vi "Periodic Tasks (Austen Adler's conflicted copy 2013-10-16).vi"(8 "error in":errorcluster) -> ()   [LabVIEW 2012]
doc: "This VI runs in parallel to other tasks. It can contain as many user-defined periodic loops as you need. These can carry out PID or other sorts of timed response."
uses:
  <vilib>/Rock Robotics/SystemInterfaces/Utilities/FPGA_UtilitiesLED Source.ctl
  <vilib>/Rock Robotics/SystemInterfaces/Utilities/FPGA_UtilitiesLED State.ctl
  <vilib>/Rock Robotics/WPI/Compressor/WPI_CompressorGetSetRefNum.vi
  <vilib>/Rock Robotics/WPI/Joystick/WPI_JoystickGetSetRefNum.vi
  Robot Global Data.vi
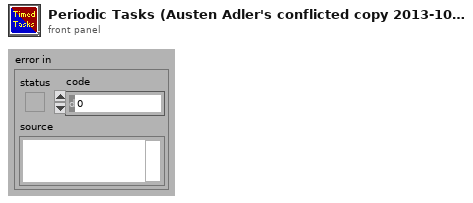
[diagram p1: front panel]
types:
  T1 = typedef "FPGA_UtilitiesLED State.ctl" = enum16{"Off", "On", "Toggle"}
  T2 = typedef "FPGA_UtilitiesLED Source.ctl" = enum16{"User LED", "FPGA LED"}
  T3 = typedef "WPI_JoystickDevRef.ctl" = cluster{"Device":T4}
  T4 = typedef "WPI_JoystickDeviceEnum.ctl" = enum16{"USB 1", "USB 2", "USB 3", "USB 4", "Kinect 1", "Kinect 2"}
  T5 = typedef "WPI_JoystickButtonState.ctl" = cluster{"Button 1":bool, "Button 2":bool, "Button 3":bool, "Button 4":bool, "Button 5":bool, "Button 6":bool, "Button 7":bool, "Button 8":bool, "Button 9":bool, "Button 10":bool, "Button 11":bool, "Button 12":bool}
  T6 = typedef "WPI_CompressorDevRef.ctl" = cluster{"DevStatus":errorcluster, "DigitalInputDevRef":T7, "RelayDevRef":T10}
  T7 = typedef "WPI_DigitalInputDevRef.ctl" = cluster{"DevStatus":errorcluster, "DIO Channel":T8, "Digital Module":T9}
  T8 = typedef "FPGA_DIOChannel.ctl" = enum8{"DIO 1", "DIO 2", "DIO 3", "DIO 4", "DIO 5", "DIO 6", "DIO 7", "DIO 8", "DIO 9", "DIO 10", "DIO 11", "DIO 12", "DIO 13", "DIO 14", "Invalid"}
  T9 = typedef "FPGA_TypedefDigitalModule.ctl" = enum16{"Digital Module 1", "Digital Module 2"}
  T10 = typedef "WPI_RelayDevRef.ctl" = cluster{"DevStatus":errorcluster, "Relay Channel":T11, "Digital Module":T9, "Relay Direction":T12}
  T11 = typedef "FPGA_DIORelayChannel.ctl" = enum8{"Relay 1", "Relay 2", "Relay 3", "Relay 4", "Relay 5", "Relay 6", "Relay 7", "Relay 8", "Invalid"}
  T12 = typedef "WPI_RelayDirection.ctl" = enum16{"Both directions", "Forward only", "Reverse only"}
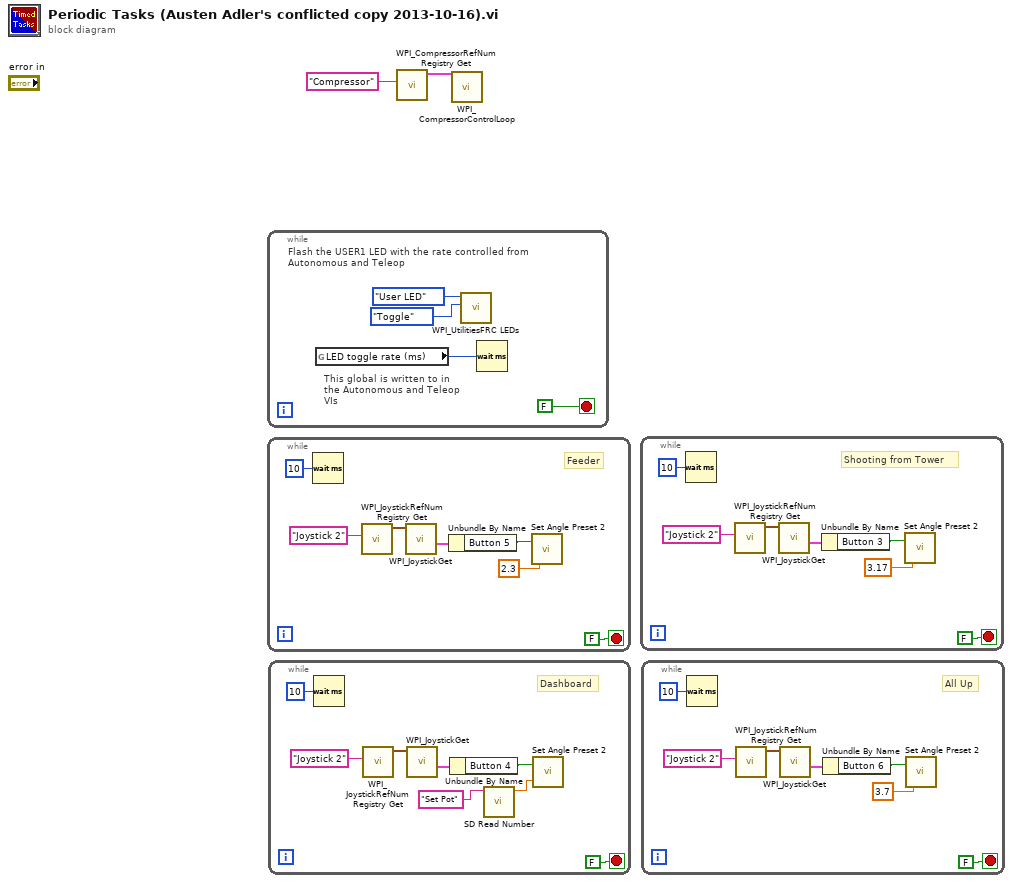
[diagram p0: block diagram]
diagram:
  n1 = while {
    stop <- FALSE stop-if-true
    # "This global is written to in the Autonomous and Teleop VIs"
    # "Flash the USER1 LED with the rate controlled from Autonomous and Teleop"
    n2 = global read "Robot Global Data.vi" "LED toggle rate (ms)"() -> (w3:u32)
    n3 = call <vilib>:"WPI_UtilitiesFRC LEDs.vi"("State"=FPGA_UtilitiesLED_State."Toggle", "LED Type"=FPGA_UtilitiesLED_Source."User LED") -> ()  [unwired: 1 in, 9 out]
    n4 = Wait (ms)(milliseconds to wait=w3) -> ()  [unwired: 1 out]
  }
  n5 = while {
    stop <- FALSE stop-if-true
    # "Feeder"
    n6 = Wait (ms)(milliseconds to wait=u32 10) -> ()  [unwired: 1 out]
    n7 = call <vilib>:"WPI_JoystickRefNum Registry Get.vi"("refnum name"="Joystick 2") -> ("JoystickDevRef"=w13:T3)  [unwired: 1 in, 9 out]
    n8 = call <vilib>:"WPI_JoystickGet.vi"("JoystickDevRef"=w13) -> ("Buttons"=w10:T5)  [unwired: 1 in, 5 out]
    n9 = Unbundle By Name(w10) -> ("Button 5"=w8:bool)
    n10 = call "Set Angle Preset 2.vi"("Set Angle"=2.3, "Enable"=w8) -> ()  [unwired: 1 in]
  }
  n11 = while {
    stop <- FALSE stop-if-true
    # "Dashboard"
    n12 = Wait (ms)(milliseconds to wait=u32 10) -> ()  [unwired: 1 out]
    n13 = call <vilib>:"WPI_JoystickRefNum Registry Get.vi"("refnum name"="Joystick 2") -> ("JoystickDevRef"=w21:T3)  [unwired: 1 in, 9 out]
    n14 = call <vilib>:"WPI_JoystickGet.vi"("JoystickDevRef"=w21) -> ("Buttons"=w18:T5)  [unwired: 1 in, 5 out]
    n15 = Unbundle By Name(w18) -> ("Button 4"=w16:bool)
    n16 = call <vilib>:"SD Read Number.vi"("Name"="Set Pot" ("refnum name")) -> ("Numeric"=w14:dbl)  [unwired: 8 in, 2 out]
    n17 = call "Set Angle Preset 2.vi"("Set Angle"=w14, "Enable"=w16) -> ()  [unwired: 1 in]
  }
  n18 = call <vilib>:"WPI_CompressorRefNum Registry Get.vi"("refnum name"="Compressor") -> ("CompressorDevRef"=w1:T6)  [unwired: 9 in, 1 out]
  n19 = call <vilib>:"WPI_CompressorControlLoop.vi"("CompressorDevRef"=w1) -> ()  [unwired: 11 in]
  n20 = while {
    stop <- FALSE stop-if-true
    # "Shooting from Tower"
    n21 = Wait (ms)(milliseconds to wait=u32 10) -> ()  [unwired: 1 out]
    n22 = call <vilib>:"WPI_JoystickRefNum Registry Get.vi"("refnum name"="Joystick 2") -> ("JoystickDevRef"=w28:T3)  [unwired: 1 in, 9 out]
    n23 = call <vilib>:"WPI_JoystickGet.vi"("JoystickDevRef"=w28) -> ("Buttons"=w25:T5)  [unwired: 1 in, 5 out]
    n24 = Unbundle By Name(w25) -> ("Button 3"=w23:bool)
    n25 = call "Set Angle Preset 2.vi"("Set Angle"=3.17, "Enable"=w23) -> ()  [unwired: 1 in]
  }
  n26 = while {
    stop <- FALSE stop-if-true
    # "All Up"
    n27 = Wait (ms)(milliseconds to wait=u32 10) -> ()  [unwired: 1 out]
    n28 = call <vilib>:"WPI_JoystickRefNum Registry Get.vi"("refnum name"="Joystick 2") -> ("JoystickDevRef"=w35:T3)  [unwired: 1 in, 9 out]
    n29 = call <vilib>:"WPI_JoystickGet.vi"("JoystickDevRef"=w35) -> ("Buttons"=w32:T5)  [unwired: 1 in, 5 out]
    n30 = Unbundle By Name(w32) -> ("Button 6"=w30:bool)
    n31 = call "Set Angle Preset 2.vi"("Set Angle"=3.7, "Enable"=w30) -> ()  [unwired: 1 in]
  }
